vi "Update Pin Map from File.vi"(8 "error in (no error)":errorcluster, 10 "pin map path":path) -> (0 "error out":errorcluster, 2 "pin map id":string)   [LabVIEW 2020, in "MeasurementLink TestStand Integration.lvlib"]
doc: "Updates the pin map service with the contents of the file specified by <b>pin map path</b>."
uses:
  MeasurementLink TestStand Integration.lvlib
  MeasurementLink Pin Map Client/RPC Messages/ni_measurementlink_pinmap_v1_UpdatePinMapFromXmlRequest.ctl
  MeasurementLink gRPC Utilities/gRPC Client Pool/FGV Action.ctl
  MeasurementLink Pin Map Client/MeasurementLink Pin Map Client.lvlib
  MeasurementLink gRPC Utilities/gRPC Client Pool/gRPC Client Pool.lvclass
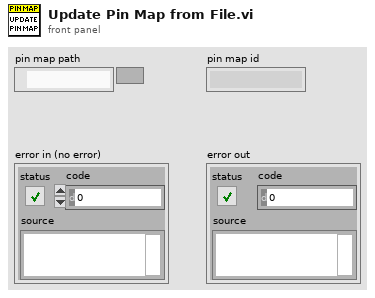
[diagram p1: front panel]
types:
  T1 = typedef "MeasurementLink gRPC Utilities.lvlib/gRPC Client Pool.lvclass/FGV Action.ctl" = enum16{"Get Discovery Client", "Get Session Client", "Get Pinmap Client", "Destroy Clients"}
  T2 = typedef "MeasurementLink Pin Map Client.lvlib/ni_measurementlink_pinmap_v1_UpdatePinMapFromXmlRequest.ctl" = cluster{"pin_map_id":string, "pin_map_xml":string}
  T3 = typedef "grpc-lvsupport-release.lvlib/grpcId.ctl" = u64
  T4 = typedef "MeasurementLink Pin Map Client.lvlib/ni_measurementlink_pinmap_v1_PinMap.ctl" = cluster{"pin_map_id":string}
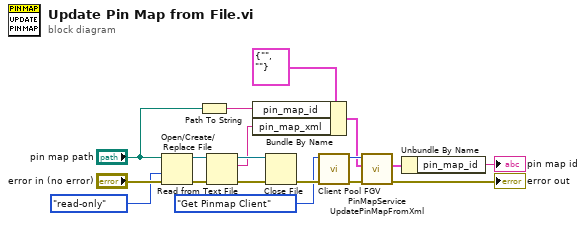
[diagram p0: block diagram]
diagram:
  n1 = Open/Create/Replace File(file path (use dialog)="pin map path", error in="error in (no error)", access (0:read/write)=enum16{"read/write", "read-only", "write-only"}."read-only") -> (refnum out=w6:refnum<file>, error out=w5:errorcluster)  [unwired: 3 in, 1 out]
  n2 = Path To String(path="pin map path") -> (string=w3:string)
  n3 = Read from Text File(file (use dialog)=w6, error in=w5) -> (refnum out=w9:refnum<file>, text=w7:string, error out=w8:errorcluster)  [unwired: 2 in, 1 out]
  n4 = Bundle By Name(cluster=T2 {"pin_map_id"="", "pin_map_xml"=""} ("Request Data"), "pin_map_id"=w3, "pin_map_xml"=w7) -> (w11:T2)
  n5 = Close File(refnum=w9, error in=w8) -> (error out=w15:errorcluster)  [unwired: 1 out]
  n6 = call "Client Pool FGV.vi"("error in (no error)"=w15, "Action"=FGV_Action."Get Pinmap Client") -> ("error out"=w16:errorcluster, "grpc client id"=w14:T3)  [unwired: 8 in]
  n7 = call "PinMapService UpdatePinMapFromXml.vi"("error in"=w16, "Request Data"=w11, "gRPC ID"=w14) -> ("error out"=→"error out":errorcluster, "Response Data"=w12:T4)  [unwired: 6 in, 1 out]
  n8 = Unbundle By Name(w12) -> ("pin_map_id"=→"pin map id":string)
